vi "_PC_RTcheck instrument_type.vi"(8 "error in (no error)":errorcluster) -> (0 "error out":errorcluster)   [LabVIEW 2018]
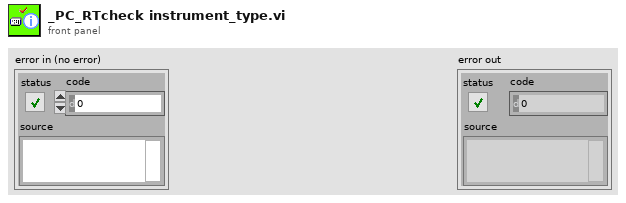
[diagram p1: front panel]
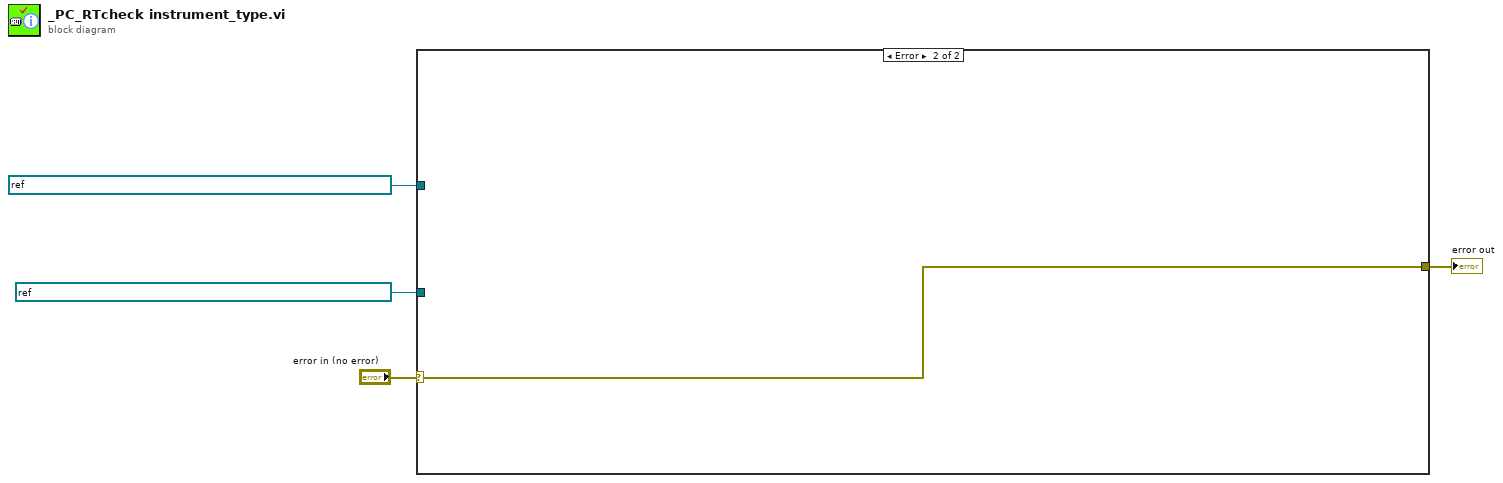
[diagram p0: block diagram]
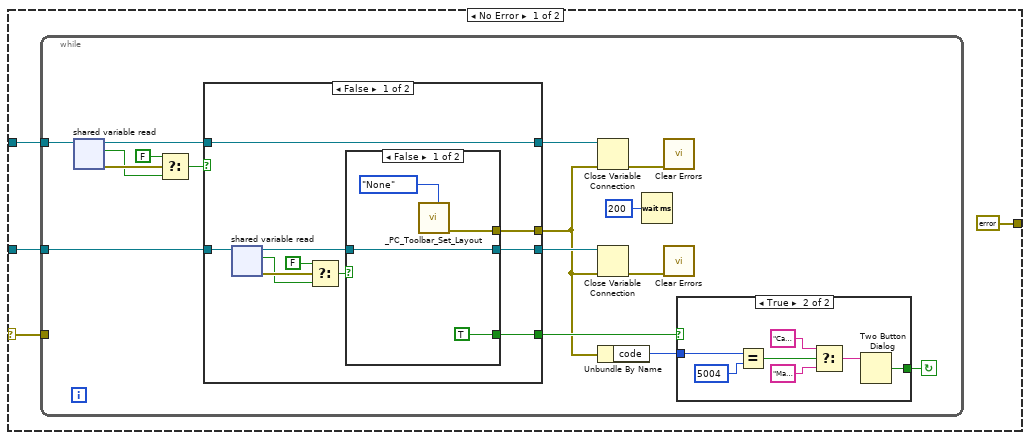
[diagram p2: hidden frame]
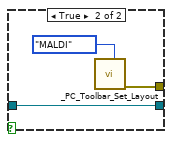
[diagram p3: hidden frame]
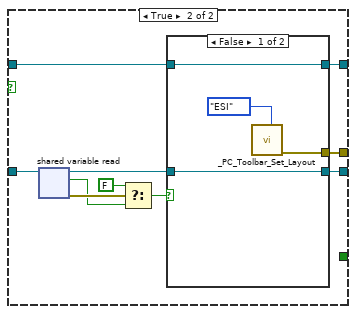
[diagram p4: hidden frame]
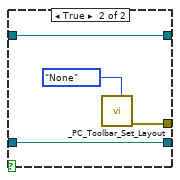
[diagram p5: hidden frame]
diagram:
  n1 = case shown="Error" "error in (no error)" {
    selector: "error in (no error)" -> [w5 w67]
    tunnel: [errorcluster {"status"=FALSE, "code"=0, "source"=""} ("error IO") w67] -> w4
    tunnel: refnum<k21> "ni.var.psp://NI-sbRIO/_RT_CtrlLoop_Laser_Variables/LaserExist" ("shared variable refnum in") -> [w7 _]
    tunnel: refnum<k21> "ni.var.psp://NI-sbRIO/_RT_CtrlLoop_D999_Variables/D999_Exist" ("shared variable refnum in") -> [w6 _]
    frame No Error {
      n2 = while {
        tunnel: w7 -> [w17]
        tunnel: w6 -> [w16]
        tunnel: w5 -> [_]
        stop <- w23 continue-if-true
        n3 = shared-variable-read(w16) -> (w18:refnum<k21>, w15:errorcluster, w14:bool)  [unwired: 1 in]
        n4 = Select(t=FALSE, s=w15, f=w14) -> (s? t:f=w12:bool)
        n5 = case shown="False" w12 {
          tunnel: [w34 _] -> w24
          tunnel: w17 -> [w33 w51]
          tunnel: [w31 w49] -> w20
          tunnel: w18 -> [w30 w48]
          tunnel: [w30 w47] -> w21
          tunnel: [w25 w46] -> w11
          frame False {
            n6 = shared-variable-read(w33) -> (w32:refnum<k21>, w28:errorcluster, w27:bool)  [unwired: 1 in]
            n7 = Select(t=FALSE, s=w28, f=w27) -> (s? t:f=w26:bool)
            n8 = case shown="False" w26 {
              tunnel: [TRUE _] -> w34
              tunnel: w32 -> [w37 w40]
              tunnel: [w37 w40] -> w31
              tunnel: [w35 w39] -> w25
              frame False {
                n9 = call "_PC_Toolbar_Set_Layout.vi"("MachineType"=enum16{"None", "MALDI", "ESI"}."None") -> ("error out"=w35:errorcluster)  [unwired: 10 in]
              }
              frame True {
                n10 = call "_PC_Toolbar_Set_Layout.vi"("MachineType"=enum16{"None", "MALDI", "ESI"}."MALDI") -> ("error out"=w39:errorcluster)  [unwired: 10 in]
              }
            }
          }
          frame True {
            n11 = shared-variable-read(w51) -> (w50:refnum<k21>, w44:errorcluster, w43:bool)  [unwired: 1 in]
            n12 = Select(t=FALSE, s=w44, f=w43) -> (s? t:f=w42:bool)
            n13 = case shown="False" w42 {
              tunnel: w50 -> [w54 w58]
              tunnel: [w54 w58] -> w49
              tunnel: w48 -> [w53 w57]
              tunnel: [w53 w57] -> w47
              tunnel: [w52 w56] -> w46
              frame False {
                n14 = call "_PC_Toolbar_Set_Layout.vi"("MachineType"=enum16{"None", "MALDI", "ESI"}."ESI") -> ("error out"=w52:errorcluster)  [unwired: 10 in]
              }
              frame True {
                n15 = call "_PC_Toolbar_Set_Layout.vi"("MachineType"=enum16{"None", "MALDI", "ESI"}."None") -> ("error out"=w56:errorcluster)  [unwired: 10 in]
              }
            }
          }
        }
        n16 = Close Variable Connection(8:w11, 11:w21) -> (0:w9:errorcluster)
        n17 = Close Variable Connection(8:w11, 11:w20) -> (0:w10:errorcluster)
        n18 = Unbundle By Name(w11) -> ("code"=w19:i32)
        n19 = Wait (ms)(milliseconds to wait=u32 200) -> ()  [unwired: 1 out]
        n20 = call <vilib>:"Clear Errors.vi"("error in (no error)"=w9) -> ()  [unwired: 5 in, 2 out]
        n21 = call <vilib>:"Clear Errors.vi"("error in (no error)"=w10) -> ()  [unwired: 5 in, 2 out]
        n22 = case shown="True" w24 {
          tunnel: [_ w66] -> w23
          tunnel: w19 -> [_ w65]
          frame False {
          }
          frame True {
            n23 = Equal?(x=w65, y=5004) -> (x = y?=w63:bool)
            n24 = Select(t="Can't Find Firmware.\nRecheck?", s=w63, f="Machine type check error.\nRecheck?" ("message")) -> (s? t:f=w60:string)
            n25 = Two Button Dialog(message=w60) -> (T button?=w66:bool)  [unwired: 2 in]
          }
        }
      }
    }
    frame Error {
    }
  }
  "error out" <- w4
